vi "PixyI2C_Parser.vi"(5 "Array":dbl[](array[numeric]), 9 "Array Size":i32) -> (4 "Signature 1":bool, 6 "X Center":dbl, 8 "Y Center":dbl, 10 "Width":dbl, 15 "Height":dbl)   [LabVIEW 2016]
panel:
  out "Message Index":dbl
  # "****Please add template to this VI*******"
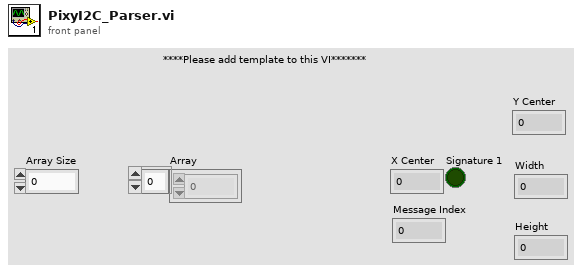
[diagram p1: front panel]
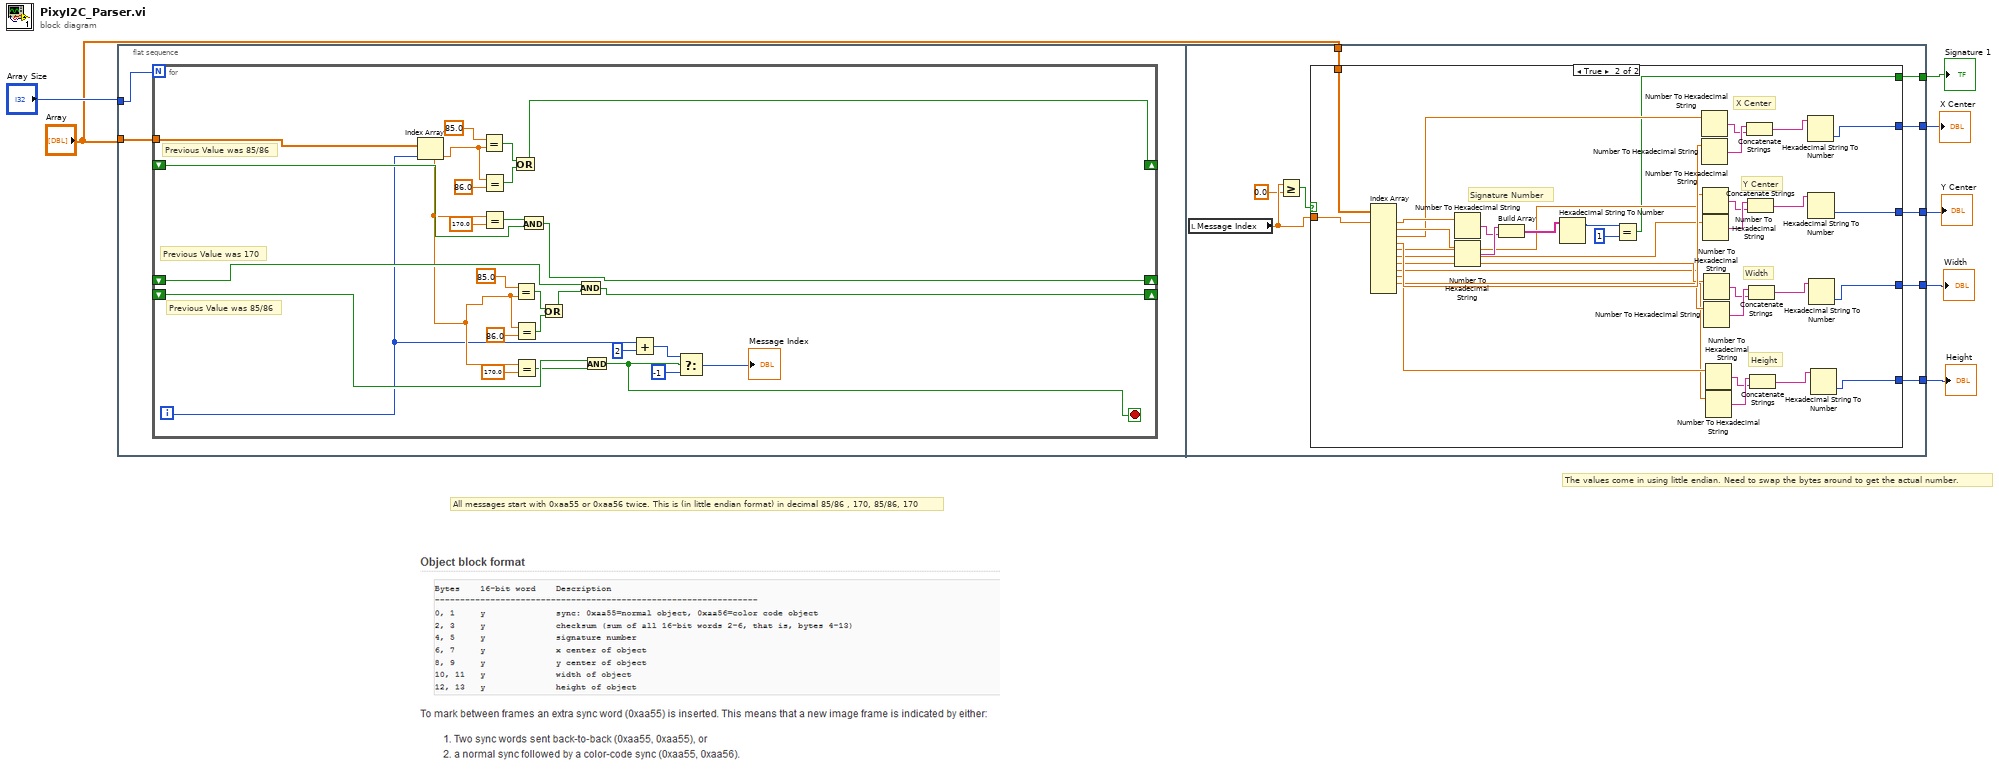
[diagram p0: block diagram]
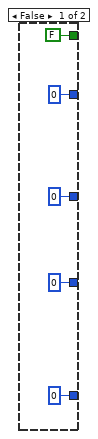
[diagram p2: hidden frame]
diagram:
  # "The values come in using little endian. Need to swap the bytes around to get the actual number."
  # "All messages start with 0xaa55 or 0xaa56 twice. This is (in little endian format) in decimal 85/86 , 170, 85/86, 170"
  n1 = flat-sequence {
    tunnel: "Array Size" -> [w9]
    tunnel: "Array" -> [w8]
    tunnel: [w42] -> w6
    tunnel: [w41] -> w5
    tunnel: [w40] -> w4
    tunnel: [w39] -> w3
    tunnel: [w38] -> w2
    tunnel: "Array" -> [w37]
    frame #0 {
      n2 = for {
        N: w9 -> [_]
        shift-right: [w32] -> _
        shift-left: _ -> [w29]
        shift-right: [w22] -> _
        shift-left: _ -> [w21]
        shift-right: [w20] -> _
        shift-left: _ -> [w19]
        tunnel: w8 -> [w10]
        i -> [w12]
        stop <- w11 stop-if-true
        # "Previous Value was 85/86"
        # "Previous Value was 170"
        # "Previous Value was 85/86"
        n3 = Index Array(array=w10, index=w12) -> (element=w17:dbl)
        n4 = Equal?(x=85.0, y=w17) -> (x = y?=w33:bool)
        n5 = Equal?(x=w17, y=86.0) -> (x = y?=w34:bool)
        n6 = Equal?(x=w17, y=170.0) -> (x = y?=w30:bool)
        n7 = Or(x=w33, y=w34) -> (x .or. y?=w32:bool)
        n8 = Equal?(x=85.0, y=w17) -> (x = y?=w24:bool)
        n9 = Equal?(x=w17, y=86.0) -> (x = y?=w23:bool)
        n10 = Equal?(x=w17, y=170.0) -> (x = y?=w18:bool)
        n11 = And(x=w30, y=w29) -> (x .and. y?=w22:bool)
        n12 = Or(x=w24, y=w23) -> (x .or. y?=w25:bool)
        n13 = And(x=w21, y=w25) -> (x .and. y?=w20:bool)
        n14 = And(x=w19, y=w18) -> (x .and. y?=w11:bool)
        n15 = Add(x=w12, y=2) -> (x+y=w16:i32)
        n16 = Select(t=w16, s=w11, f=-1) -> (s? t:f=→"Message Index":i32)
      }
    }
    frame #1 {
      n17 = local read "Message Index"() -> (w45:dbl)
      n18 = Greater Or Equal?(x=w45, y=0.0) -> (x >= y?=w43:bool)
      n19 = case shown="True" w43 {
        tunnel: w37 -> [_ w84]
        tunnel: w45 -> [_ w82]
        tunnel: [u32 0 w67] -> w42
        tunnel: [u32 0 w66] -> w41
        tunnel: [u32 0 w65] -> w40
        tunnel: [u32 0 w64] -> w39
        tunnel: [FALSE w51] -> w38
        frame False {
        }
        frame True {
          # "Height"
          # "Width"
          # "Y Center"
          # "X Center"
          # "Signature Number"
          n20 = Index Array(array=w84, index #1=w82) -> (element #1=w83:dbl, element #2=w81:dbl, element #3=w75:dbl, element #4=w74:dbl, element #5=w73:dbl, element #6=w72:dbl, element #7=w71:dbl, element #8=w70:dbl, element #9=w69:dbl, element #10=w68:dbl)  [unwired: 10 in, 1 out]
          n21 = Number To Hexadecimal String(2:w83) -> (0:w79:string)  [unwired: 1 in]
          n22 = Number To Hexadecimal String(2:w81) -> (0:w80:string)  [unwired: 1 in]
          n23 = Build Array(w80, w79) -> (w78:string[])
          n24 = Hexadecimal String To Number(string=w78) -> (offset past number=w77:i32)  [unwired: 2 in, 1 out]
          n25 = Equal?(x=w77, y=1) -> (x = y?=w51:bool)
          n26 = Number To Hexadecimal String(2:w75) -> (0:w62:string)  [unwired: 1 in]
          n27 = Number To Hexadecimal String(2:w74) -> (0:w63:string)  [unwired: 1 in]
          n28 = Number To Hexadecimal String(2:w73) -> (0:w59:string)  [unwired: 1 in]
          n29 = Number To Hexadecimal String(2:w72) -> (0:w60:string)  [unwired: 1 in]
          n30 = Number To Hexadecimal String(2:w71) -> (0:w56:string)  [unwired: 1 in]
          n31 = Number To Hexadecimal String(2:w70) -> (0:w57:string)  [unwired: 1 in]
          n32 = Number To Hexadecimal String(2:w69) -> (0:w53:string)  [unwired: 1 in]
          n33 = Number To Hexadecimal String(2:w68) -> (0:w54:string)  [unwired: 1 in]
          n34 = Concatenate Strings(w63, w62) -> (w61:string)
          n35 = Concatenate Strings(w60, w59) -> (w58:string)
          n36 = Concatenate Strings(w57, w56) -> (w55:string)
          n37 = Concatenate Strings(w54, w53) -> (w52:string)
          n38 = Hexadecimal String To Number(string=w61) -> (number=w67:u32)  [unwired: 2 in, 1 out]
          n39 = Hexadecimal String To Number(string=w58) -> (number=w66:u32)  [unwired: 2 in, 1 out]
          n40 = Hexadecimal String To Number(string=w55) -> (number=w65:u32)  [unwired: 2 in, 1 out]
          n41 = Hexadecimal String To Number(string=w52) -> (number=w64:u32)  [unwired: 2 in, 1 out]
        }
      }
    }
  }
  "Y Center" <- w5
  "Width" <- w4
  "Height" <- w3
  "X Center" <- w6
  "Signature 1" <- w2
